vi "Initialise Config Folder Path.vi"(8 "error in (no error)":errorcluster) -> (0 "error out":errorcluster, 1 "Config files folder found?":bool, 3 "Config Files Folder Path":path)   [LabVIEW 2013]
uses:
  Global Variables/General Globals.vi
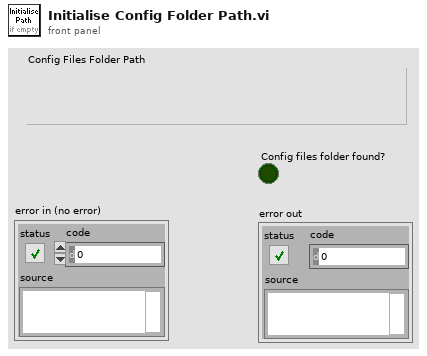
[diagram p1: front panel]
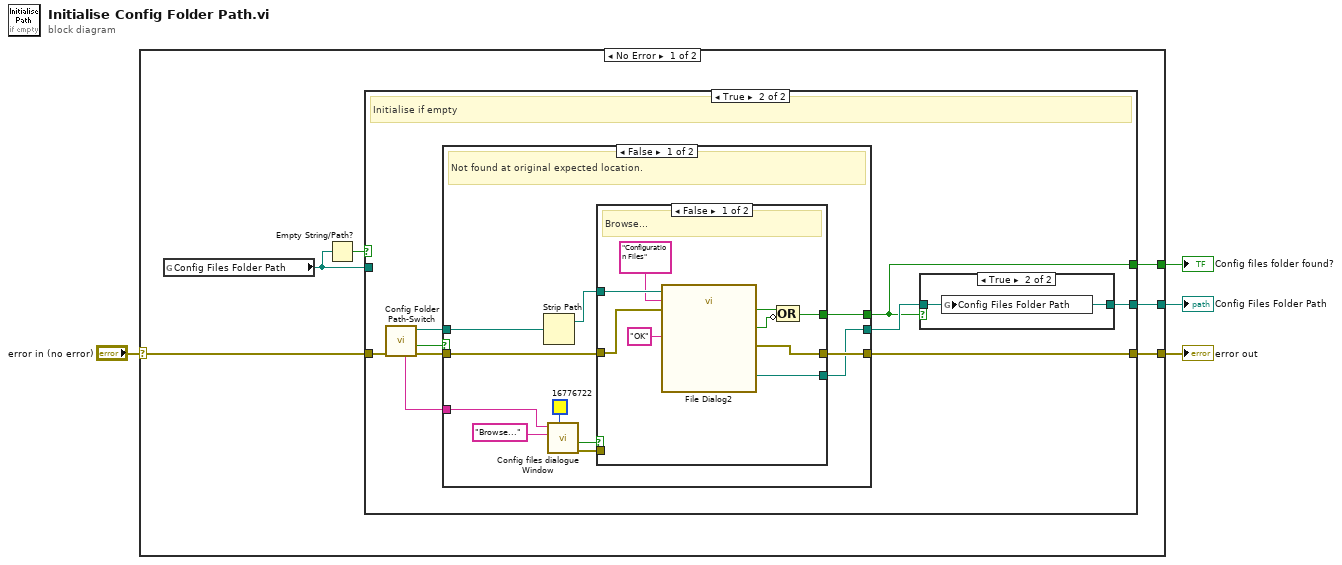
[diagram p0: block diagram]
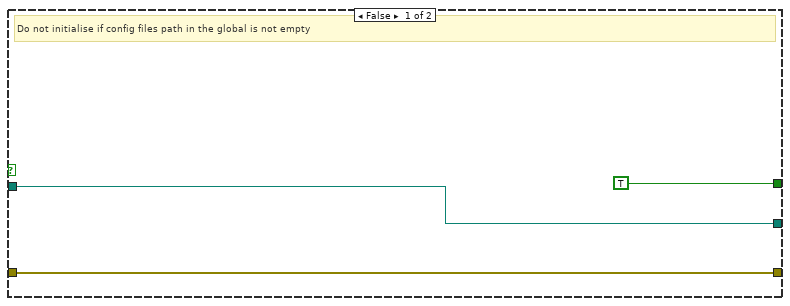
[diagram p2: hidden frame]
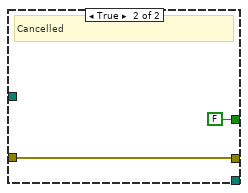
[diagram p4: hidden frame]
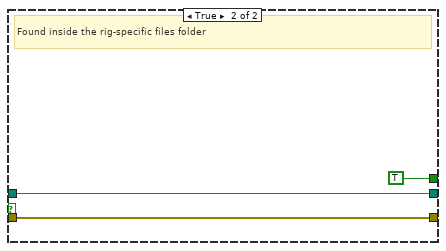
[diagram p5: hidden frame]
diagram:
  n1 = case shown="No Error" "error in (no error)" {
    selector: "error in (no error)" -> [w10 w49]
    tunnel: [w9 w49] -> w4
    tunnel: [w8 _] -> w2
    tunnel: [w7 _] -> w1
    frame No Error {
      n2 = global read "General Globals.vi" "Config Files Folder Path"() -> (w5:path)
      n3 = Empty String/Path?(string/path=w5) -> (empty?=w6:bool)
      n4 = case shown="True" w6 {
        tunnel: w10 -> [w11 w22]
        tunnel: [w11 w19] -> w9
        tunnel: [TRUE ("file or folder exists?") w16] -> w8
        tunnel: [w12 w15] -> w7
        tunnel: w5 -> [w12 _]
        frame False {
          # "Do not initialise if config files path in the global is not empty"
        }
        frame True {
          # "Initialise if empty"
          n5 = call "Config Folder Path-Switch.vi"("error in (no error)"=w22) -> ("error out"=w20:errorcluster, "file or folder exists?"=w21:bool, "dup path"=w17:path, "Message string"=w14:string)  [unwired: 6 in, 1 out]
          n6 = case shown="False" w21 {
            tunnel: w20 -> [w34 w48]
            tunnel: [w33 w48] -> w19
            tunnel: [w32 w47] -> w18
            tunnel: [w31 TRUE ("file or folder exists?")] -> w16
            tunnel: w17 -> [w30 w47]
            tunnel: w14 -> [w29 _]
            frame False {
              # "Not found at original expected location."
              n7 = Strip Path(path=w30) -> (stripped path=w28:path)  [unwired: 1 out]
              n8 = call "Config files dialogue Window.vi"("Colour"=u32 16776722, "Caption-Right button (OK)"="Browse...", "Message string"=w29) -> ("error out"=w24:errorcluster, "Cancelled (Left button pressed)"=w25:bool)  [unwired: 7 in]
              n9 = case shown="False" w25 {
                tunnel: w34 -> [w43 w44]
                tunnel: [w42 w44] -> w33
                tunnel: [w40 _] -> w32
                tunnel: [w37 FALSE] -> w31
                tunnel: w28 -> [w36 _]
                tunnel: w24 -> [_ _]
                frame False {
                  # "Browse..."
                  n10 = call "File Dialog2"("start path"=w36, "button label"="OK", "default name"="Configuration Files", "error in"=w43) -> ("selected path"=w40:path, "exists"=w39:bool, "cancelled"=w38:bool, "error out"=w42:errorcluster)  [unwired: 8 in]
                  n11 = Compound Arithmetic op=OR(w39, invert w38) -> (w37:bool)
                }
                frame True {
                  # "Cancelled"
                }
              }
            }
            frame True {
              # "Found inside the rig-specific files folder"
            }
          }
          n12 = case shown="True" w16 {
            tunnel: w18 -> [_ w23]
            tunnel: [_ w23] -> w15
            frame False {
            }
            frame True {
              n13 = global write "General Globals.vi" "Config Files Folder Path"(w23) -> ()
            }
          }
        }
      }
    }
    frame Error {
    }
  }
  "error out" <- w4
  "Config Files Folder Path" <- w1
  "Config files folder found?" <- w2
